vi "Get VI Index.vi"(11 "Parsed Results Data (by VI)":T1) -> (3 "row":i32)   [LabVIEW 2019]
uses:
  <vilib>/addons/analyzer/_vianresshared.llb/VIAnRes Parsed Results Data (by VI).ctl
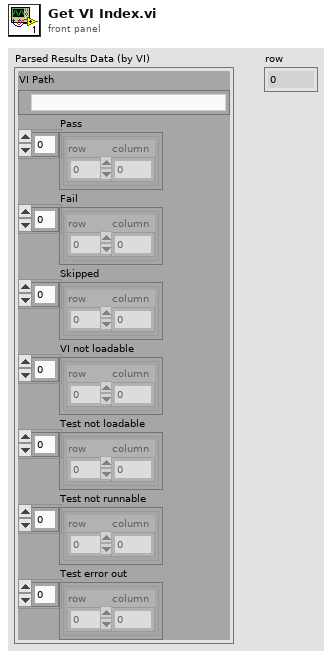
[diagram p1: front panel]
types:
  T1 = typedef "VIAnRes Parsed Results Data (by VI).ctl" = cluster{"VI Path":path, "Pass":cluster{"row":i32, "column":i32}[], "Fail":cluster{"row":i32, "column":i32}[], "Skipped":cluster{"row":i32, "column":i32}[], "VI not loadable":cluster{"row":i32, "column":i32}[], "Test not loadable":cluster{"row":i32, "column":i32}[], "Test not runnable":cluster{"row":i32, "column":i32}[], "Test error out":cluster{"row":i32, "column":i32}[]}
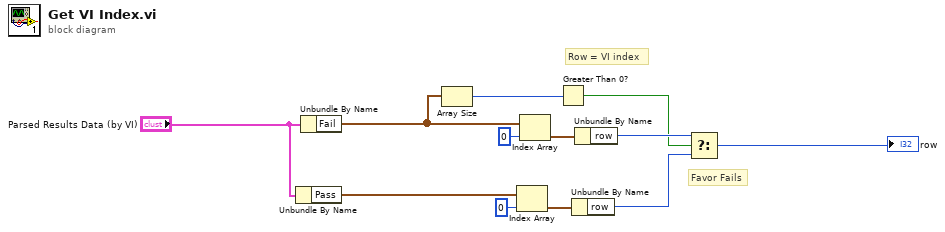
[diagram p0: block diagram]
diagram:
  # "Row = VI index"
  # "Favor Fails"
  n1 = Unbundle By Name("Parsed Results Data (by VI)") -> ("Pass"=w6:cluster{"row":i32, "column":i32}[])
  n2 = Unbundle By Name("Parsed Results Data (by VI)") -> ("Fail"=w7:cluster{"row":i32, "column":i32}[])
  n3 = Array Size(array=w7) -> (size(s)=w8:i32)
  n4 = Index Array(array=w6, index=0) -> (element=w4:cluster{"row":i32, "column":i32})
  n5 = Index Array(array=w7, index=0) -> (element=w1:cluster{"row":i32, "column":i32})
  n6 = Greater Than 0?(x=w8) -> (x > 0?=w9:bool)
  n7 = Unbundle By Name(w4) -> ("row"=w11:i32)
  n8 = Unbundle By Name(w1) -> ("row"=w10:i32)
  n9 = Select(t=w10, s=w9, f=w11) -> (s? t:f=→"row":i32)
